vi "mod_Add pilot tone.vi"(0 "input":cdb[](array[numeric]), 5 "pilot tone frequency (normalized)":dbl, 7 "starting phase (radians)":dbl, 9 "pilot tone amplitude":dbl=1.0, 11 "error in (no error)":errorcluster, 13 "reset? (T)":bool=TRUE) -> (4 "input+pilot tone":cdb[](array[numeric]), 15 "error out":errorcluster)   [LabVIEW 2020, in "niAMT.lvlib"]
uses:
  <vilib>/addons/Modulation/niAMT.lvlib
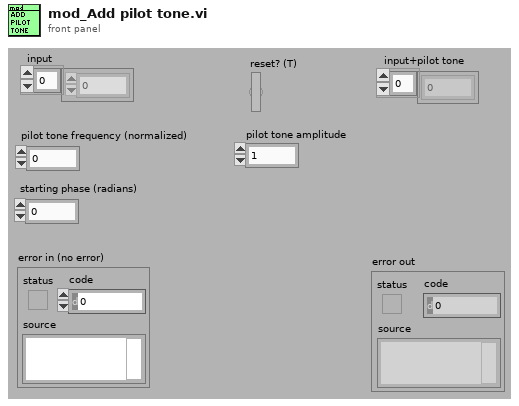
[diagram p1: front panel]
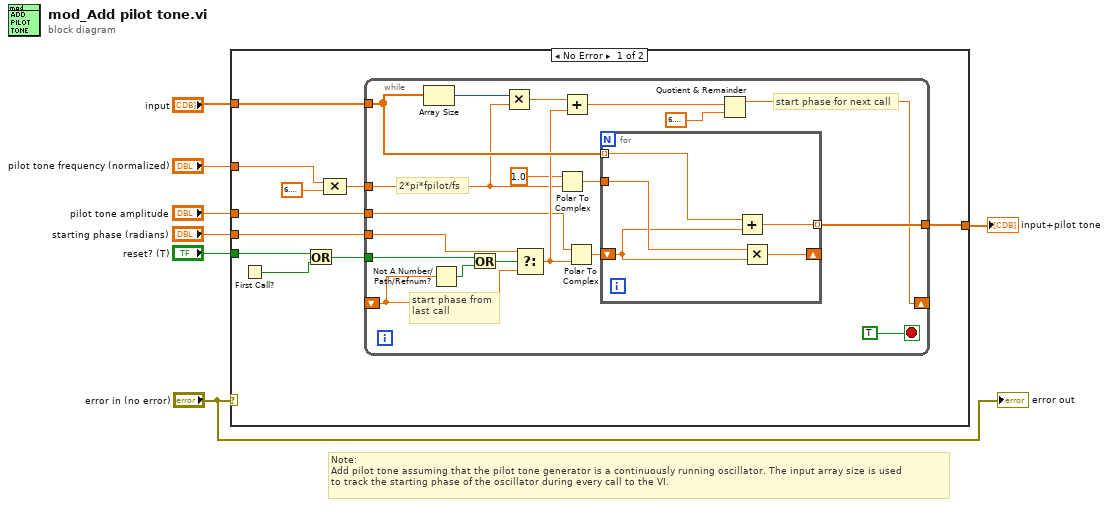
[diagram p0: block diagram]
diagram:
  # "Note:\nAdd pilot tone assuming that the pilot tone generator is a continuously running oscillator. The input array size is used\nto track the starting phase of the oscillator during every call to the VI."
  n1 = case shown="No Error" "error in (no error)" {
    tunnel: "pilot tone amplitude" -> [w13 _]
    tunnel: "input" -> [w12 _]
    tunnel: "pilot tone frequency (normalized)" -> [w11 _]
    tunnel: "starting phase (radians)" -> [w10 _]
    tunnel: "reset? (T)" -> [w9 _]
    tunnel: [w8 _] -> w2
    frame No Error {
      n2 = First Call?() -> (First Call?: T/F=w15:bool)
      n3 = Or(x=w9, y=w15) -> (x .or. y?=w14:bool)
      n4 = Compound Arithmetic op=MULTIPLY(w11, 6.283185307179586) -> (w16:dbl)
      n5 = while {
        tunnel: w16 -> [w19]
        tunnel: w10 -> [w34]
        tunnel: w13 -> [w32]
        tunnel: w12 -> [w35]
        shift-right: [w23] -> _
        shift-left: _ -> [w27]
        tunnel: w14 -> [w25]
        tunnel: [w28] -> w8
        stop <- TRUE stop-if-true
        # "2*pi*fpilot/fs"
        # "start phase for next call"
        # "start phase from\nlast call"
        n6 = Array Size(array=w35) -> (size(s)=w20:i32)
        n7 = Not A Number/Path/Refnum?(number/path/refnum=w27) -> (NaN/Path/Refnum?=w26:bool)
        n8 = Or(x=w25, y=w26) -> (x .or. y?=w24:bool)
        n9 = Multiply(x=w20, y=w19) -> (x*y=w21:dbl)
        n10 = Select(t=w34, s=w24, f=w27) -> (s? t:f=w33:dbl)
        n11 = Polar To Complex(1:w19, 2:1.0 ("r")) -> (0:w29:cdb)
        n12 = Add(x=w21, y=w33) -> (x+y=w18:dbl)
        n13 = Polar To Complex(1:w33, 2:w32) -> (0:w31:cdb)
        n14 = for {
          tunnel: w35 -> [w41] mode=indexing
          shift-right: [w37] -> _
          shift-left: w31 -> [w38]
          tunnel: w29 -> [w39]
          tunnel: [w40] -> w28 mode=indexing
          n15 = Add(x=w41, y=w38) -> (x+y=w40:cdb)
          n16 = Multiply(x=w39, y=w38) -> (x*y=w37:cdb)
        }
        n17 = Quotient & Remainder(x=w18, y=6.283185307179586) -> (x-y*floor(x/y)=w23:dbl)  [unwired: 1 out]
      }
    }
    frame Error {
    }
  }
  "input+pilot tone" <- w2
  "error out" <- "error in (no error)"
